vi "CalcScore.vi"(9 ">HitTime>":u32, 10 "Combo":u32, 11 "OldScore":u32) -> (3 "NewScore":u32)   [LabVIEW 2022 SP3]
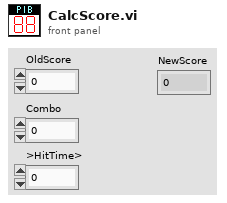
[diagram p1: front panel]
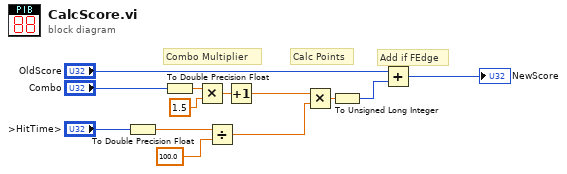
[diagram p0: block diagram]
diagram:
  # "Add if FEdge"
  # "Calc Points"
  # "Combo Multiplier"
  n1 = To Double Precision Float(number=">HitTime>") -> (double precision float=w4:dbl)
  n2 = To Double Precision Float(number="Combo") -> (double precision float=w10:dbl)
  n3 = Multiply(x=w10, y=1.5) -> (x*y=w8:dbl)
  n4 = Divide(x=w4, y=100.0) -> (x/y=w1:dbl)
  n5 = Increment(x=w8) -> (x+1=w2:dbl)
  n6 = Multiply(x=w2, y=w1) -> (x*y=w6:dbl)
  n7 = To Unsigned Long Integer(number=w6) -> (unsigned 32bit integer=w11:u32)
  n8 = Add(x="OldScore", y=w11) -> (x+y=→"NewScore":u32)
